vi "Decorate.vi"(7 "Actor":refnum<class "Actor.lvclass">, 11 "Actor":refnum<class "Actor.lvclass">) -> (5 "Actor":refnum<class "Actor.lvclass">)   [LabVIEW 2020, in "_Template.lvlib" / "{{Actor}}.lvlib" / "Actor.lvclass"]
uses:
  Actor.lvclass
  Actor.lvclass/Actor.ctl
  jettl/jettl/Actor/Actor.lvclass
panel:
  # "This front panel should not be manipulated."
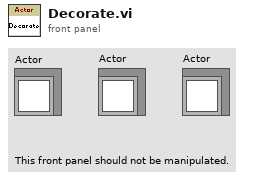
[diagram p1: front panel]
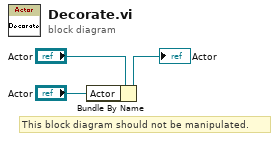
[diagram p0: block diagram]
diagram:
  # "This block diagram should not be manipulated."
  n1 = Bundle By Name(cluster="Actor", "Actor"="Actor") -> (→"Actor":refnum<class "Actor.lvclass">)
